vi "Inficon - Load metal parameters.vi"(8 "Error In":errorcluster, 10 "Material refnum":refnum<vi>) -> (0 "Error Out":errorcluster, 2 "Evaporator parameters":T1={"Rise Time 1 [mm:ss]"=0.0, "Soak Power 1 [%]"=0.0, "Soak Time 1 [mm:ss]"=0.0, "Rise Time 2 [mm:ss]"=0.0, "Soak Power 2 [%]"=0.0, "Soak Time 2 [mm:ss]"=0.0, "Shutter Delay"=enum."No", "New Rate"=0.0, "Rate Ramp Time [mm:ss]"=0.0, "Idle Ramp [mm:ss]"=0.0, "Idle Power [%]"=0.0, "Time Power"=enum."No", "Xtal Switch S"=0, "Xtal Switch Q"=0, "Tool Factor 1"=10.0, "Tool Factor 2"=10.0, "Deposition Rate [Å/s]"=0.0, "Final Thickness [kÅ]"=0.0, "Thickness Spt [kÅ]"=0.0, "Density [g/cm3]"=0.5, "Z-Ratio"=0.1, "Sensor"=1, "Source"=1, "Crucible"=1, "Control Gain [%]"=0.1, "Control TC [s]"=0.1, "Control DT [s] 2"=0.1, "Max Power"=0.1, "Sample"=1, "Hold Time [mm:ss]"=0.0} {"Hold Time [mm:ss]" min=0.0 max=5999.0 format="%<%M:%S>t"; "Sample" max=99 step=1; "Max Power" min=0.0 max=100.0 step=0.1 format="%.;%.1f"; "Control DT [s] 2" min=0.1 max=100.0 step=0.1 format="%.;%.1f"; "Control TC [s]" min=0.1 max=100.0 step=0.1 format="%.;%.1f"; "Control Gain [%]" min=0.01 max=99.99 step=0.01 format="%.;%.3f"; "Crucible" max=8 step=1; "Source" min=1 max=2 step=1; "Sensor" min=1 max=2 step=1; "Z-Ratio" min=0.1 max=9.999 step=0.001 format="%.;%.3f"; "Density [g/cm3]" min=0.5 max=99.99 step=0.01 format="%.;%.2f"; "Thickness Spt [kÅ]" min=0.0 max=999.0 step=0.001 format="%.;%.3f"; "Final Thickness [kÅ]" min=0.0 max=999.0 step=0.001 format="%.;%.3f"; "Deposition Rate [Å/s]" min=0.0 max=999.9 step=0.1 format="%.;%.1f"; "Tool Factor 2" min=10.0 max=500.0 step=0.1 format="%.;%.1f"; "Tool Factor 1" min=10.0 max=500.0 step=0.1 format="%.;%.1f"; "Xtal Switch Q" max=9 step=1; "Xtal Switch S" max=9 step=1; "Idle Power [%]" min=0.0 max=100.0 step=0.1 format="%.;%.1f"; "Idle Ramp [mm:ss]" min=0.0 max=5999.0 format="%<%M:%S>t"; "Rate Ramp Time [mm:ss]" min=0.0 max=5999.0 format="%<%M:%S>t"; "New Rate" min=0.0 max=999.9 step=0.1 format="%.;%.1f"; "Soak Time 2 [mm:ss]" min=0.0 max=5999.0 format="%<%M:%S>t"; "Soak Power 2 [%]" min=0.0 max=100.0 step=0.1 format="%.;%.1f"; "Soak Time 1 [mm:ss]" min=0.0 max=5999.0 format="%<%M:%S>t"; "Rise Time 2 [mm:ss]" min=0.0 max=5999.0 format="%<%M:%S>t"; "Soak Power 1 [%]" min=0.0 max=100.0 step=0.1 format="%.;%.1f"; "Rise Time 1 [mm:ss]" min=0.0 max=5999.0 format="%<%M:%S>t"})   [LabVIEW 2014]
uses:
  <vilib>/Utility/xml.llb/Read From XML File(string).vi
  Typedef/Inficon - Evaporator parameters.ctl
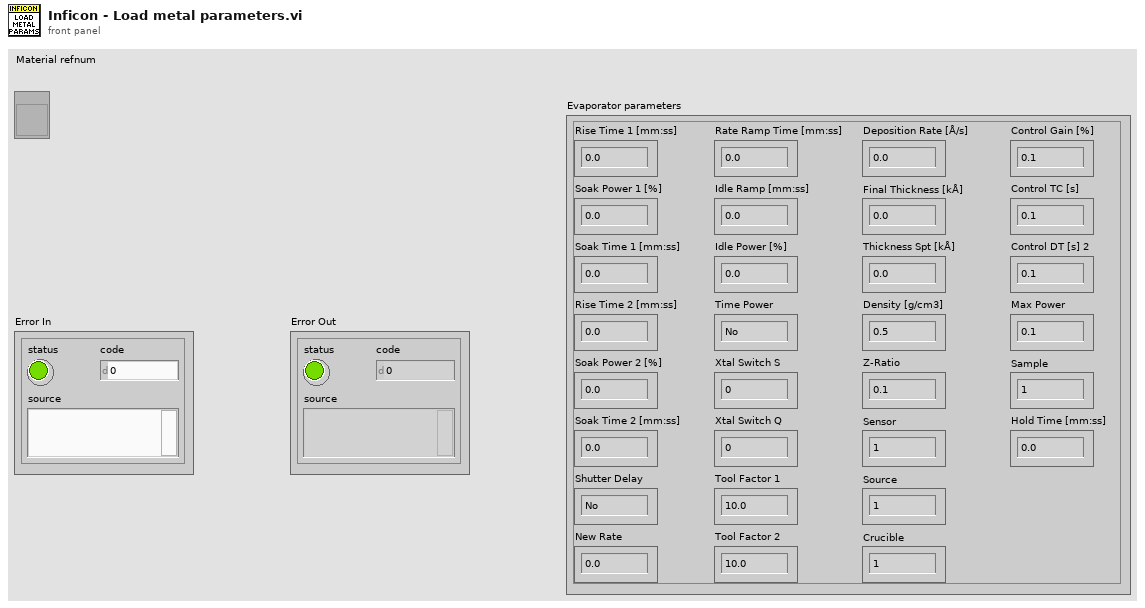
[diagram p1: front panel]
types:
  T1 = typedef "Inficon - Evaporator parameters.ctl" = cluster{"Rise Time 1 [mm:ss]":dbl, "Soak Power 1 [%]":dbl, "Soak Time 1 [mm:ss]":dbl, "Rise Time 2 [mm:ss]":dbl, "Soak Power 2 [%]":dbl, "Soak Time 2 [mm:ss]":dbl, "Shutter Delay":enum16{"No", "Yes"}, "New Rate":dbl, "Rate Ramp Time [mm:ss]":dbl, "Idle Ramp [mm:ss]":dbl, "Idle Power [%]":dbl, "Time Power":enum16{"No", "Yes"}, "Xtal Switch S":u8, "Xtal Switch Q":u8, "Tool Factor 1":dbl, "Tool Factor 2":dbl, "Deposition Rate [Å/s]":dbl, "Final Thickness [kÅ]":dbl, "Thickness Spt [kÅ]":dbl, "Density [g/cm3]":dbl, "Z-Ratio":dbl, "Sensor":u8, "Source":u8, "Crucible":u8, "Control Gain [%]":dbl, "Control TC [s]":dbl, "Control DT [s] 2":dbl, "Max Power":dbl, "Sample":u8, "Hold Time [mm:ss]":dbl}
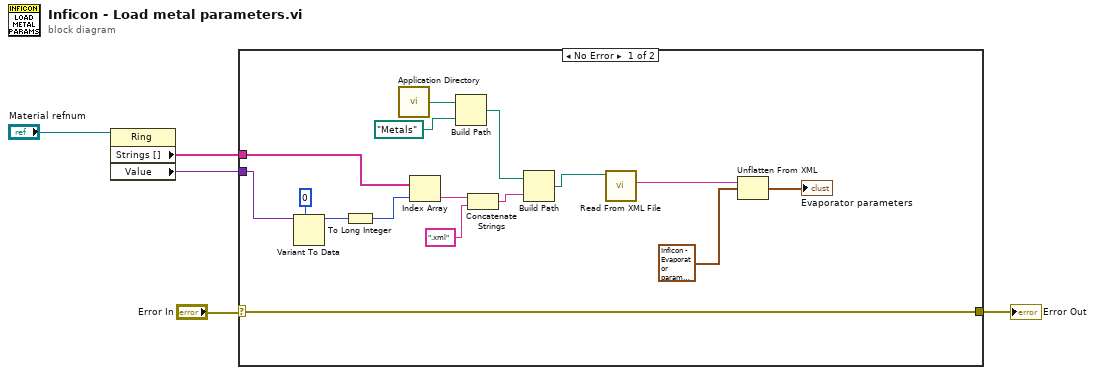
[diagram p0: block diagram]
diagram:
  n1 = property class="Ring"(reference="Material refnum") -> ("Strings []"=w2:string[], "Value"=w1:variant)  [unwired: 1 in, 2 out]
  n2 = case shown="No Error" "Error In" {
    selector: "Error In" -> [w18 w22]
    tunnel: [w18 w22] -> w4
    tunnel: w2 -> [w9 _]
    tunnel: w1 -> [w8 _]
    frame No Error {
      n3 = Variant To Data(type=u16 0, Variant=w8) -> (data=w6:u16)  [unwired: 1 in, 1 out]
      n4 = To Long Integer(number=w6) -> (32bit integer=w19:i32)
      n5 = call <vilib>:"Application Directory.vi"() -> ("Application Directory"=w14:path)
      n6 = Index Array(array=w9, index=w19) -> (element=w17:string)
      n7 = Build Path(base path=w14, name or relative path=path "Metals") -> (appended path=w12:path)
      n8 = Concatenate Strings(w17, ".xml" ("string")) -> (w16:string)
      n9 = Build Path(base path=w12, name or relative path=w16) -> (appended path=w21:path)
      n10 = call-poly <vilib>:"Read From XML File.vi"("XML File Path"=w21) -> ("XML Elements"=w20:string)  [unwired: 8 in, 2 out]
      n11 = Unflatten From XML(xml string=w20, type=T1 {"Rise Time 1 [mm:ss]"=0.0, "Soak Power 1 [%]"=0.0, "Soak Time 1 [mm:ss]"=0.0, "Rise Time 2 [mm:ss]"=0.0, "Soak Power 2 [%]"=0.0, "Soak Time 2 [mm:ss]"=0.0, "Shutter Delay"=enum."No", "New Rate"=0.0, "Rate Ramp Time [mm:ss]"=0.0, "Idle Ramp [mm:ss]"=0.0, "Idle Power [%]"=0.0, "Time Power"=enum."No", "Xtal Switch S"=0, "Xtal Switch Q"=0, "Tool Factor 1"=10.0, "Tool Factor 2"=10.0, "Deposition Rate [Å/s]"=0.0, "Final Thickness [kÅ]"=0.0, "Thickness Spt [kÅ]"=0.0, "Density [g/cm3]"=0.5, "Z-Ratio"=0.1, "Sensor"=1, "Source"=1, "Crucible"=1, "Control Gain [%]"=0.1, "Control TC [s]"=0.1, "Control DT [s] 2"=0.1, "Max Power"=0.1, "Sample"=1, "Hold Time [mm:ss]"=0.0} ("Evaporator parameters")) -> (value=→"Evaporator parameters":T1)  [unwired: 1 in, 1 out]
    }
    frame Error {
    }
  }
  "Error Out" <- w4
